vi "Read Adapters Info Registry2.vi"(8 "error in (no error)":errorcluster, 10 "Array in":string[](array[string]), 11 "Numeric":i32) -> (0 "error out":errorcluster, 3 "Array out":string[](array[string]))   [LabVIEW 2017]
uses:
  <vilib>/registry/registry.llb/Registry RtKey.ctl
  <vilib>/registry/registry.llb/Registry SAM.ctl
  <vilib>/registry/registry.llb/Read Registry Value Simple STR.vi
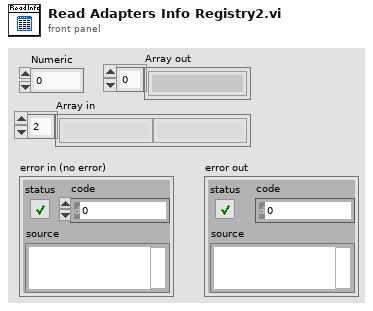
[diagram p1: front panel]
types:
  T1 = typedef "Registry SAM.ctl" = enum32{"KEY_QUERY_VALUE", "KEY_SET_VALUE", "KEY_CREATE_SUB_KEY", "KEY_ENUMERATE_SUB_KEYS", "KEY_NOTIFY", "KEY_CREATE_LINK", "KEY_READ", "KEY_WRITE", "KEY_ALL_ACCESS", "KEY_READ | KEY_WRITE"}
  T2 = typedef "Registry RtKey.ctl" = enum32{"HKEY_CLASSES_ROOT", "HKEY_CURRENT_USER", "HKEY_LOCAL_MACHINE", "HKEY_USERS", "HKEY_PERFORMANCE_DATA", "HKEY_CURRENT_CONFIG", "HKEY_DYN_DATA"}
  T3 = typedef "Registry refnum.ctl" = refnum<k1>
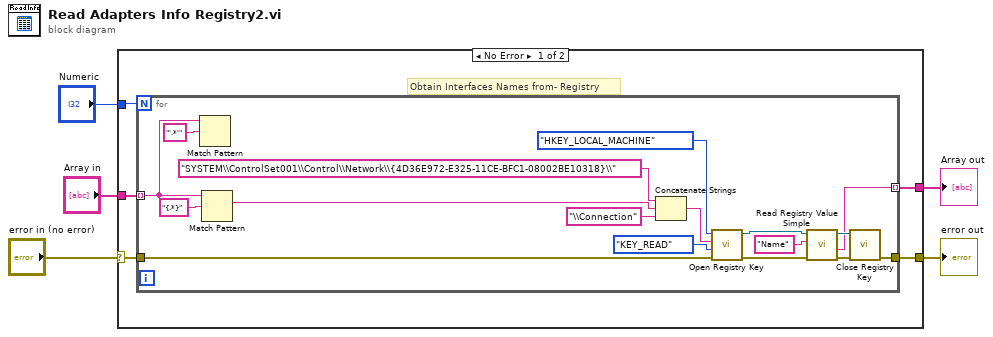
[diagram p0: block diagram]
diagram:
  n1 = case shown="No Error" "error in (no error)" {
    selector: "error in (no error)" -> [w7 w28]
    tunnel: "Array in" -> [w10 _]
    tunnel: "Numeric" -> [w9 _]
    tunnel: [w8 w28] -> w4
    tunnel: [w6 _] -> w1
    frame No Error {
      # "Obtain Interfaces Names from- Registry"
      n2 = for {
        N: w9 -> [_]
        tunnel: w10 -> [w15] mode=indexing
        tunnel: w7 -> [w12]
        tunnel: [w11] -> w8
        tunnel: [w13] -> w6 mode=indexing
        n3 = Match Pattern(string=w15, regular expression="'.*'") -> ()  [unwired: 1 in, 4 out]
        n4 = Match Pattern(string=w15, regular expression="{.*}") -> (match substring=w14:string)  [unwired: 1 in, 3 out]
        n5 = Concatenate Strings("SYSTEM\\ControlSet001\\Control\\Network\\{4D36E972-E325-11CE-BFC1-08002BE10318}\\" ("subkey"), w14, "\\Connection" ("string")) -> (w19:string)
        n6 = call <vilib>:"Open Registry Key.vi"("error in (no error)"=w12, "security access mask (KEY_READ | KEY_WRITE)"=Registry_SAM."KEY_READ", "subkey"=w19, "root key (HKEY_LOCAL_MACHINE)"=Registry_RtKey."HKEY_LOCAL_MACHINE") -> ("error out"=w25:errorcluster, "refnum out"=w21:T3)  [unwired: 6 in]
        n7 = call-poly <vilib>:"Read Registry Value Simple.vi"("error in (no error)"=w25, "value"="Name", "refnum"=w21) -> ("error out"=w24:errorcluster, "String/Binary data"=w13:string, "refnum out"=w16:T3)  [unwired: 3 in, 1 out]
        n8 = call <vilib>:"Close Registry Key.vi"("error in (no error)"=w24, "refnum"=w16) -> ("error out"=w11:errorcluster)  [unwired: 5 in]
      }
    }
    frame Error {
    }
  }
  "error out" <- w4
  "Array out" <- w1
